vi "templates FIELDS data keys.vi"(7 "HTM Keys":T1, 8 "error in (no error)":errorcluster, 10 "Template Keys":T1, 11 "Connection Refnum":T2) -> (0 "error out":errorcluster, 3 "Connection Refnum":T2, 5 "HTM Keys":T1)   [LabVIEW 2011]
uses:
  Addons/internet/utils/keyedarr.llb/Keyed Array.ctl
  SI.LIB/ODBC/SQL Controls/Connection Refnum.ctl
  Addons/internet/utils/strutil.llb/Case Matching.ctl
  server/database/Fields/Field Order By.ctl
  server/database/Fields/Field Record.ctl
  server/database/Fields/Field DataTypes.ctl
  server/database/Fields/Field NextItem.ctl
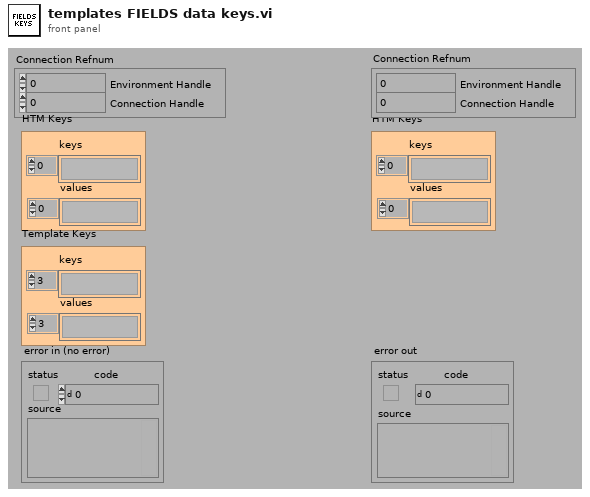
[diagram p1: front panel]
types:
  T1 = typedef "Keyed Array.ctl" = cluster{"keys":string[], "values":string[]}
  T2 = typedef "Connection Refnum.ctl" = cluster{"Environment Handle":i32, "Connection Handle":i32}
  T3 = typedef "Field Record.ctl" = cluster{"ixField":i32, "iSequenceOrder":i32, "sxFieldId":string, "sxSequenceId":string, "sDisplayName":string, "sValue":string, "sUnits":string, "nDataType":T4, "nNextItem":T5, "fSystem":bool, "fSystemValue":bool, "fRequired":bool, "fSetAtTest":bool, "fTestField":bool, "fDeleted":bool, "fIndexed":bool, "fFreeList":bool}
  T4 = typedef "Field DataTypes.ctl" = enum32{"text", "numeric", "list", "timestamp", "boolean"}
  T5 = typedef "Field NextItem.ctl" = enum32{"Reset", "Retain", "Auto-Increment"}
  T6 = typedef "Field Order By.ctl" = enum32{"sxSequenceId", "sxFieldId", "sDisplayName", "sValue", "fSetAtTest", "fRequired", "nNextItem"}
  T7 = typedef "Case Matching.ctl" = enum16{"a != A", "a == A", "system"}
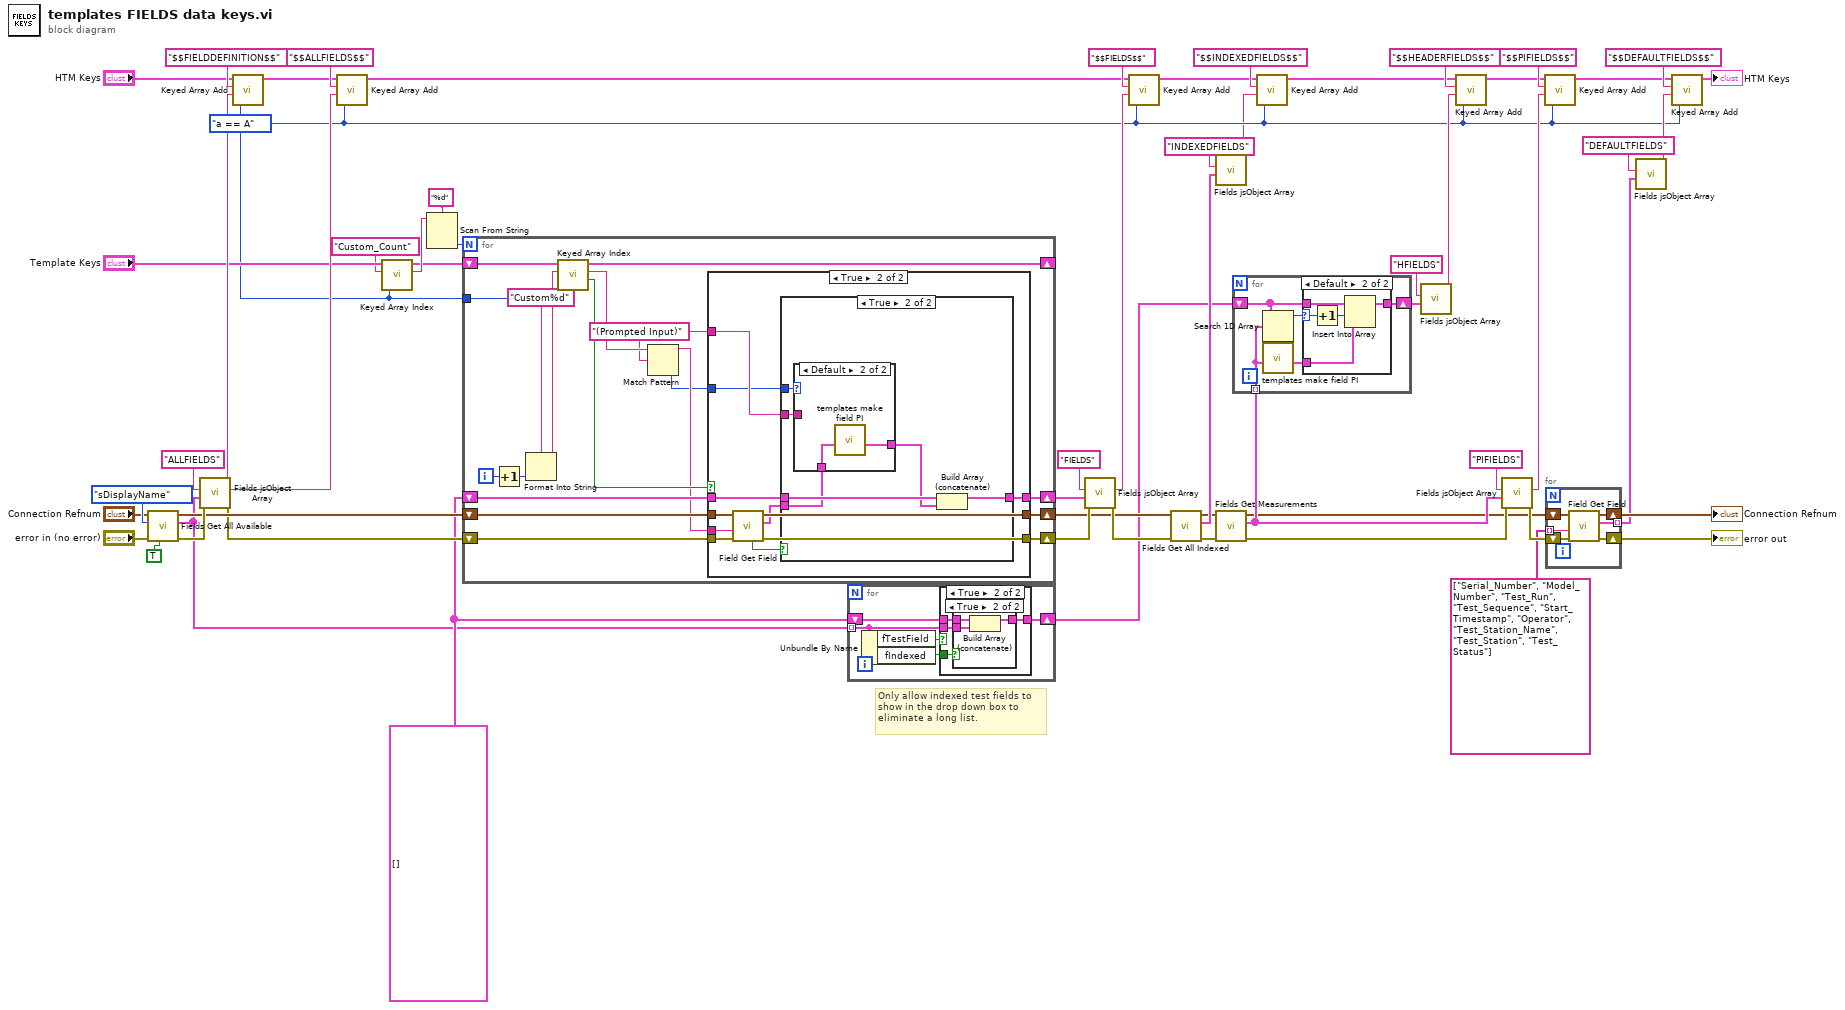
[diagram p0: block diagram]
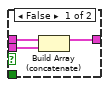
[diagram p2: hidden frame]
diagram:
  w7 = T3[] []
  w14 = Case_Matching."a == A" ("case matching (sensitive)")
  # "Only allow indexed test fields to\nshow in the drop down box to\neliminate a long list."
  n1 = call "Fields Get All Available.vi"("Combine All? (f)"=TRUE, "error in (no error)"="error in (no error)", "Sort by (sxSequenceId)"=Field_Order_By."sDisplayName", "Connection Refnum"="Connection Refnum") -> ("error out"=w52:errorcluster, "System or ALL Combined Fields"=w6:T3[], "Connection Refnum"=w41:T2)  [unwired: 1 in, 4 out]
  n2 = call "Fields jsObject Array.vi"("error in (no error)"=w52, "FIELDS (none)"=w6, "Fields jsObject Array Name (\"FIELDS\")"="ALLFIELDS") -> ("error out"=w40:errorcluster, "Fields jsObject Array"=w53:string, "Field jsObject Definition"=w54:string)  [unwired: 1 in, 5 out]
  n3 = call "Keyed Array Add.vi"("case matching (sensitive)"=w14, "value"=w54, "key"="$$FIELDDEFINITION$$", "array in"="HTM Keys") -> ("array out"=w55:T1)  [unwired: 3 out]
  n4 = call "Keyed Array Add.vi"("case matching (sensitive)"=w14, "value"=w53, "key"="$$ALLFIELDS$$", "array in"=w55) -> ("array out"=w48:T1)  [unwired: 3 out]
  n5 = call "Keyed Array Index.vi"("case matching (sensitive)"=w14, "key"="Custom_Count", "array in"="Template Keys") -> ("value"=w44:string, "duplicate array"=w42:T1)  [unwired: 1 in, 2 out]
  n6 = Scan From String(format string="%d", input string=w44) -> (output 1=w43:i32)  [unwired: 2 in, 4 out]
  n7 = for {
    N: w43 -> [_]
    shift-right: [w78] -> _
    shift-left: w42 -> [w79]
    tunnel: w14 -> [w77]
    shift-right: [w70] -> w16
    shift-left: w41 -> [w73]
    shift-right: [w71] -> w38
    shift-left: w40 -> [w72]
    shift-right: [w69] -> w8
    shift-left: w7 -> [w66]
    i -> [w75]
    w63 = "(Prompted Input)"
    n8 = Increment(x=w75) -> (x+1=w68:i32)
    n9 = Format Into String(format string="Custom%d", w68) -> (resulting string=w74:string)  [unwired: 2 in, 1 out]
    n10 = call "Keyed Array Index.vi"("case matching (sensitive)"=w77, "key"=w74, "array in"=w79) -> ("valid key"=w67:bool, "value"=w65:string, "duplicate array"=w78:T1)  [unwired: 1 in, 1 out]
    n11 = Match Pattern(string=w65, regular expression=w63) -> (before substring=w64:string, offset past match=w62:i32)  [unwired: 3 out]
    n12 = case shown="True" w67 {
      tunnel: w73 -> [w82 w93]
      tunnel: w72 -> [w81 w92]
      tunnel: [w81 w91] -> w71
      tunnel: [w82 w90] -> w70
      tunnel: w64 -> [_ w89]
      tunnel: [w80 w86] -> w69
      tunnel: w66 -> [w80 w87]
      tunnel: w63 -> [_ w84]
      tunnel: w62 -> [_ w83]
      frame False {
      }
      frame True {
        n13 = call "Field Get Field.vi"("error in (no error)"=w92, "sFieldId or sDisplayName (\"\")"=w89, "Connection Refnum"=w93) -> ("error out"=w91:errorcluster, "Field"=w88:T3, "Connection Refnum"=w90:T2, "Data Present?"=w85:bool)  [unwired: 2 in, 3 out]
        n14 = case shown="True" w85 {
          tunnel: w88 -> [_ w95]
          tunnel: w87 -> [w94 w100]
          tunnel: [w94 w99] -> w86
          tunnel: w84 -> [_ w98]
          tunnel: w83 -> [_ w96]
          frame False {
          }
          frame True {
            n15 = case shown="Default" w96 {
              tunnel: w98 -> [_ _]
              tunnel: [w101 w102] -> w97
              tunnel: w95 -> [w101 w103]
              frame -1 {
              }
              frame Default {
                n16 = call "templates make field PI.vi"("Field Information  2"=w103) -> ("Field Information"=w102:T3)  [unwired: 10 out]
              }
            }
            n17 = Build Array (concatenate)(w100, w97) -> (w99:T3[])
          }
        }
      }
    }
  }
  n18 = for {
    shift-right: [w105] -> w5
    shift-left: w7 -> [w106]
    tunnel: w6 -> [w104] mode=indexing
    n19 = Unbundle By Name(w104) -> ("fTestField"=w108:bool, "fIndexed"=w107:bool)
    n20 = case shown="True" w108 {
      tunnel: w107 -> [_ w115]
      tunnel: w106 -> [w111 w114]
      tunnel: [w110 w112] -> w105
      tunnel: w104 -> [w109 w113]
      frame False {
        n21 = Build Array (concatenate)(w111, w109) -> (w110:T3[])
      }
      frame True {
        n22 = case shown="True" w115 {
          tunnel: w114 -> [w116 w119]
          tunnel: w113 -> [_ w118]
          tunnel: [w116 w117] -> w112
          frame False {
          }
          frame True {
            n23 = Build Array (concatenate)(w119, w118) -> (w117:T3[])
          }
        }
      }
    }
  }
  n24 = call "Fields jsObject Array.vi"("error in (no error)"=w38, "FIELDS (none)"=w8, "Fields jsObject Array Name (\"FIELDS\")"="FIELDS") -> ("error out"=w18:errorcluster, "Fields jsObject Array"=w37:string)  [unwired: 1 in, 6 out]
  n25 = call "Keyed Array Add.vi"("case matching (sensitive)"=w14, "value"=w37, "key"="$$FIELDS$$", "array in"=w48) -> ("array out"=w12:T1)  [unwired: 3 out]
  n26 = call "Fields Get All Indexed.vi"("error in (no error)"=w18, "Connection Refnum"=w16) -> ("error out"=w17:errorcluster, "Fields Out"=w11:T3[], "Connection Refnum"=w4:T2)  [unwired: 7 in]
  n27 = call "Fields jsObject Array.vi"("FIELDS (none)"=w11, "Fields jsObject Array Name (\"FIELDS\")"="INDEXEDFIELDS") -> ("Fields jsObject Array"=w9:string)  [unwired: 2 in, 7 out]
  n28 = call "Fields Get Measurements.vi"("error in (no error)"=w17, "Connection Refnum"=w4) -> ("error out"=w2:errorcluster, "Measurement Fields"=w3:T3[], "dup Connection Refnum"=w1:T2)  [unwired: 1 in, 6 out]
  n29 = for {
    shift-right: [w123] -> w19
    shift-left: w5 -> [w124]
    tunnel: w3 -> [w120] mode=indexing
    n30 = Search 1D Array(1D array=w124, element=w120) -> (index of element=w121:i32)  [unwired: 1 out]
    n31 = call "templates make field PI.vi"("Field Information  2"=w120) -> ("Field Information"=w122:T3)  [unwired: 10 out]
    n32 = case shown="Default" w121 {
      selector: w121 -> [_ w126]
      tunnel: w124 -> [w125 w130]
      tunnel: [w125 w129] -> w123
      tunnel: w122 -> [_ w128]
      frame -1 {
      }
      frame Default {
        n33 = Increment(x=w126) -> (x+1=w127:i32)
        n34 = Insert Into Array(array=w130, index=w127, new element=w128) -> (w129:T3[])
      }
    }
  }
  n35 = call "Keyed Array Add.vi"("case matching (sensitive)"=w14, "value"=w9, "key"="$$INDEXEDFIELDS$$", "array in"=w12) -> ("array out"=w13:T1)  [unwired: 3 out]
  n36 = call "Fields jsObject Array.vi"("FIELDS (none)"=w19, "Fields jsObject Array Name (\"FIELDS\")"="HFIELDS") -> ("Fields jsObject Array"=w30:string)  [unwired: 2 in, 7 out]
  n37 = call "Keyed Array Add.vi"("case matching (sensitive)"=w14, "value"=w30, "key"="$$HEADERFIELDS$$", "array in"=w13) -> ("array out"=w32:T1)  [unwired: 3 out]
  n38 = call "Fields jsObject Array.vi"("error in (no error)"=w2, "FIELDS (none)"=w3, "Fields jsObject Array Name (\"FIELDS\")"="PIFIELDS") -> ("error out"=w25:errorcluster, "Fields jsObject Array"=w34:string)  [unwired: 1 in, 6 out]
  n39 = call "Keyed Array Add.vi"("case matching (sensitive)"=w14, "value"=w34, "key"="$$PIFIELDS$$", "array in"=w32) -> ("array out"=w28:T1)  [unwired: 3 out]
  n40 = for {
    shift-right: [w132] -> w23
    shift-left: w1 -> [w136]
    shift-right: [w131] -> w24
    shift-left: w25 -> [w135]
    tunnel: string[] ["Serial_Number", "Model_Number", "Test_Run", "Test_Sequence", "Start_Timestamp", "Operator", "Test_Station_Name", "Test_Station", "Test_Status"] -> [w134] mode=indexing
    tunnel: [w133] -> w21 mode=indexing
    n41 = call "Field Get Field.vi"("error in (no error)"=w135, "sFieldId or sDisplayName (\"\")"=w134, "Connection Refnum"=w136) -> ("error out"=w131:errorcluster, "Field"=w133:T3, "Connection Refnum"=w132:T2)  [unwired: 2 in, 4 out]
  }
  "error out" <- w24
  "Connection Refnum" <- w23
  n42 = call "Fields jsObject Array.vi"("FIELDS (none)"=w21, "Fields jsObject Array Name (\"FIELDS\")"="DEFAULTFIELDS") -> ("Fields jsObject Array"=w20:string)  [unwired: 2 in, 7 out]
  n43 = call "Keyed Array Add.vi"("case matching (sensitive)"=w14, "value"=w20, "key"="$$DEFAULTFIELDS$$", "array in"=w28) -> ("array out"=→"HTM Keys":T1)  [unwired: 3 out]
